vi "Page 1.vi"() -> ()   [LabVIEW 2020]
panel:
  in  "Stop":bool
  in  "Jump":bool
  out "Waveform Chart":dbl(graph)
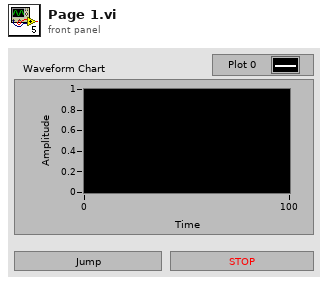
[diagram p1: front panel]
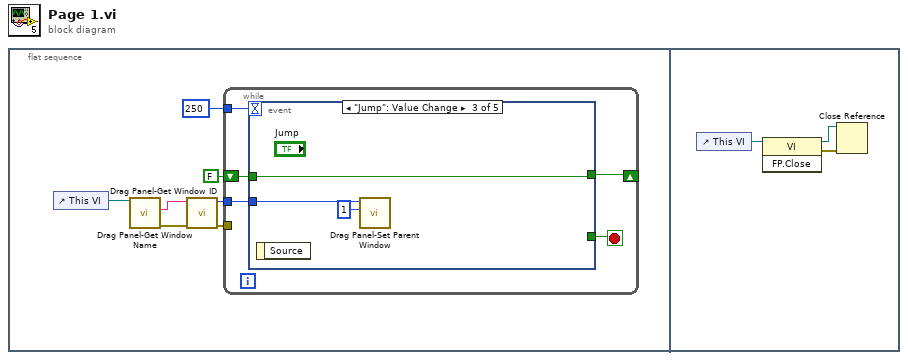
[diagram p0: block diagram]
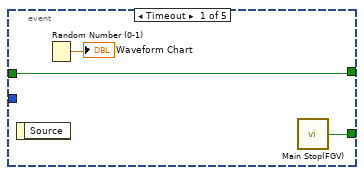
[diagram p2: hidden frame]
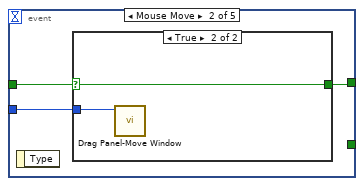
[diagram p3: hidden frame]
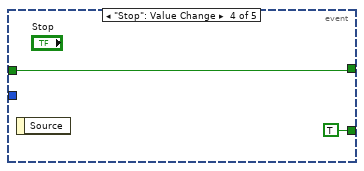
[diagram p5: hidden frame]
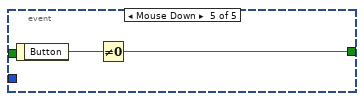
[diagram p6: hidden frame]
diagram:
  n1 = flat-sequence {
    frame #0 {
      n2 = control-ref of="This VI"() -> (w5:refnum<vi>)
      n3 = call "Drag Panel-Get Window Name.vi"("VI Refnum In"=w5) -> ("error out"=w4:errorcluster, "Window Name"=w3:string)  [unwired: 8 in, 1 out]
      n4 = call "Drag Panel-Get Window ID.vi"("error in"=w4, "Window Name"=w3) -> ("error out"=w1:errorcluster, "Window ID"=w2:u32)  [unwired: 8 in]
      n5 = while {
        tunnel: 250 -> [w12]
        shift-right: [w9] -> _
        shift-left: FALSE -> [w10]
        tunnel: w2 -> [w8]
        tunnel: w1 -> [_]
        stop <- w11 stop-if-true
        n6 = event shown="[2] \"Jump\": Value Change" {
          selector: _ -> [_ _ _ _ _]
          dyn-events: _ -> [_ _ _ _ _]
          timeout: w12 -> [_ _ _ _ _]
          tunnel: [w14 _ _ TRUE ("Stop Out") _] -> w11
          tunnel: w10 -> [w13 w18 w24 w26 _]
          tunnel: [w13 w17 w24 w26 w27] -> w9
          tunnel: w8 -> [_ w16 w23 _ _]
          event Timeout {
            n7 = event-data() -> ()  [unwired: 1 in, 1 out]
            n8 = Random Number (0-1)() -> (number: 0 to 1=→"Waveform Chart":dbl)
            n9 = call "Main Stop(FGV).vi"() -> ("Stop Out"=w14:bool)  [unwired: 4 in]
          }
          event Mouse Move {
            n10 = event-data() -> ()  [unwired: 1 in, 1 out]
            n11 = case shown="True" w18 {
              selector: w18 -> [w19 w21]
              tunnel: [w19 w21] -> w17
              tunnel: w16 -> [_ w20]
              frame False {
              }
              frame True {
                n12 = call "Drag Panel-Move Window.vi"("Window ID"=w20) -> ()  [unwired: 10 in, 1 out]
              }
            }
          }
          event "Jump": Value Change {
            n13 = event-data() -> ()  [unwired: 1 in, 1 out]
            n14 = call "Drag Panel-Set Parent Window.vi"("Parent Window ID"=u32 1, "Child Window ID"=w23) -> ()  [unwired: 8 in, 2 out]
          }
          event "Stop": Value Change {
            n15 = event-data() -> ()  [unwired: 1 in, 1 out]
          }
          event Mouse Down {
            n16 = event-data() -> ("Button"=w28:u16)  [unwired: 1 in]
            n17 = Not Equal To 0?(x=w28) -> (x != 0?=w27:bool)
          }
        }
      }
    }
    frame #1 {
      n18 = control-ref of="This VI"() -> (w31:refnum<vi>)
      n19 = invoke class="VI" method="FP.Close"(reference=w31) -> (reference out=w29:refnum<vi>, error out=w30:errorcluster)  [unwired: 2 in, 1 out]
      n20 = Close Reference(reference=w29, error in (no error)=w30) -> ()  [unwired: 1 out]
    }
  }
